vi "Upload Path.vi"(11 "Specified Path (Temp)":path=path "") -> (3 "Upload Path":path)   [LabVIEW 2020, in "HTTP Utils.lvlib"]
uses:
  HTTP Utils.lvlib
  <vilib>/Utility/sysdir.llb/System Directory Type.ctl
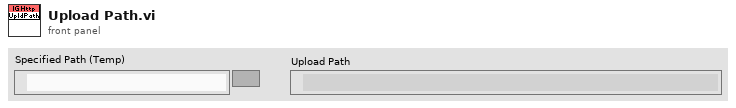
[diagram p1: front panel]
types:
  T1 = typedef "System Directory Type.ctl" = i32
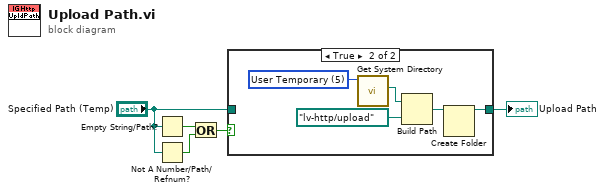
[diagram p0: block diagram]
diagram:
  n1 = Empty String/Path?(string/path="Specified Path (Temp)") -> (empty?=w5:bool)
  n2 = Not A Number/Path/Refnum?(number/path/refnum="Specified Path (Temp)") -> (NaN/Path/Refnum?=w4:bool)
  n3 = Or(x=w5, y=w4) -> (x .or. y?=w3:bool)
  n4 = case shown="True" w3 {
    tunnel: "Specified Path (Temp)" -> [w6 _]
    tunnel: [w6 w7] -> w1
    frame False {
    }
    frame True {
      w11 = T1 5 items=["User Home"=0, "User Desktop"=1, "User Documents"=2, "User Application Data"=3, "User Preferences"=4, "User Temporary"=5, "Public Documents"=6, "Public Application Data"=7, "Public Preferences"=8, "Public Cache"=13, "System Core Libraries"=9, "System Installed Libraries"=10, "Application Files"=11, "Boot Volume Root"=12] ("system directory type")
      n5 = call <vilib>:"Get System Directory.vi"("system directory type"=w11) -> ("system directory"=w10:path)  [unwired: 10 in]
      n6 = Build Path(base path=w10, name or relative path=path "lv-http/upload") -> (appended path=w8:path)
      n7 = Create Folder(path (use dialog)=w8) -> (created path=w7:path)  [unwired: 2 in, 2 out]
    }
  }
  "Upload Path" <- w1
